vi "myRIO_BRig_RT_dataExp_laser1_Tpeak.vi"() -> (2 "output_laser1_Tpeak":i32)   [LabVIEW 2014]
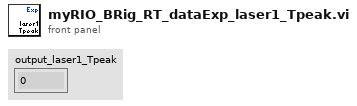
[diagram p1: front panel]
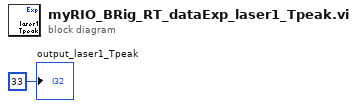
[diagram p0: block diagram]
diagram:
  "output_laser1_Tpeak" <- 33 ("output_iBlock")
